vi "Finish.vi"   [LabVIEW 2015]
doc: "This VI is called just before exiting. It is expected to close I/O refnum, save collected data, etc."
uses:
  Robot Global.vi
  <vilib>/Rock Robotics/WPI/Ultrasonic/WPI_SonarMB1010AnalogClose.vi
types:
  T1 = typedef "Robot Drive.ctl" = cluster{"RobotDriveDevRef":T2, "Joysticks":cluster{"JoystickDevRef":T10, "JoystickDevRef 2":T10}, "Sensor":T12, "Pneumatics":T31, "Defenses":cluster{"LeftArm MotorControlDeviceRef":T3, "RightArm MotorControlDeviceRef":T3}, "Hanging":cluster{"Left Erection MotorControlDeviceRef":T3, "Right Erection MotorControlDeviceRef":T3}, "Aquisition + Scoring":T35, "DigitalOutputDevRef":T39, "DigitalInputDevRef":T16}
  T2 = typedef "WPI_RobotDriveDevRef.ctl" = cluster{"DevStatus":errorcluster, "Motors[]":T3[], "Square Inputs":bool, "Max Output":dbl}
  T3 = typedef "WPI_MotorControlDeviceRef.ctl" = cluster{"DeviceStatus":errorcluster, "Type":T4, "PWM":cluster{"PWM Channel":T5, "DeadBand":T6}, "CAN":cluster{"Device Number":u8, "Control Mode":T7, "Semaphore":T8, "Max Vout":dbl, "TalonSRX Control Mode":T9}, "Invert":bool}
  T4 = typedef "WPI_MotorControlType.ctl" = enum16{"PWM", "CAN", "CANTalonSRX"}
  T5 = typedef "FPGA_DIOPWMChannel.ctl" = enum8{"PWM 0", "PWM 1", "PWM 2", "PWM 3", "PWM 4", "PWM 5", "PWM 6", "PWM 7", "PWM 8", "PWM 9", "PWM MXP 0", "PWM MXP 1", "PWM MXP 2", "PWM MXP 3", "PWM MXP 4", "PWM MXP 5", "PWM MXP 6", "PWM MXP 7", "PWM MXP 8", "PWM MXP 9", "Invalid"}
  T6 = typedef "WPI_PWMDeadband.ctl" = cluster{"Name":string, "maxPositivePwm":i32, "minPositivePwm":i32, "centerPwm":i32, "maxNegativePwm":i32, "minNegativePwm":i32, "angularRange":u16}
  T7 = typedef "WPI_CANJaguar_ControlMode.ctl" = enum8{"Percent VBus", "Current", "Speed", "Position", "Voltage"}
  T8 = typedef "Semaphore RefNum" = refnum<k1>
  T9 = typedef "WPI_CANTalonSRX_APIControlMode.ctl" = enum8{"Percent VBus", "Speed", "Position", "Slave", "Unchanged / Invalid", "Voltage Compensation", "Current", "Motion Profile"}
  T10 = typedef "WPI_JoystickDevRef.ctl" = cluster{"Device":T11}
  T11 = typedef "WPI_JoystickDeviceEnum.ctl" = enum16{"USB 0", "USB 1", "USB 2", "USB 3", "USB 4", "USB 5"}
  T12 = typedef "Sensors.ctl" = cluster{"GyroDevRef":T13, "Left Arm Limit DigitalInputDevRef":T16, "Right Arm Limit DigitalInputDevRef":T16, "Left Arm EncoderDevRef":T18, "Right Arm EncoderDevRef":T18, "Left Drive EncoderDevRef":T18, "Right Drive EncoderDevRef":T18, "BoB Photoeye DigitalInputDevRef":T16, "Range SonarMB1010AnalogDevRef":T22, "Shooter CounterDevRef":T24, "AccelerometerDevRef":T25, "Left Hanging Erecter EncoderDevRef":T18, "Right Hanging Erecter EncoderDevRef":T18, "TestDigitalInputDevRef":T16, "Shooter Counter TopDevRef":T24}
  T13 = typedef "WPI_GyroDevRef.ctl" = cluster{"DevStatus":errorcluster, "Analog Channel":T14, "Offset":dbl, "Gain (VoltsPerDegree/Second)":dbl, "Gyro Type":enum16{"Analog", "XRS450"}, "Handle":i32, "SPI Bus":T15, "Device Found":bool, "Sample Rate":dbl, "Calibrate On Open":bool}
  T14 = typedef "FPGA_AIChannel.ctl" = enum8{"AI 0", "AI 1", "AI 2", "AI 3", "AI MXP 0", "AI MXP 1", "AI MXP 2", "AI MXP 3", "Invalid"}
  T15 = typedef "spi_bus.ctl" = enum16{"SPI On-Board, CS0", "SPI On-Board, CS1", "SPI On-Board, CS2", "SPI On-Board, CS3", "SPI MXP", "Invalid"}
  T16 = typedef "WPI_DigitalInputDevRef.ctl" = cluster{"DevStatus":errorcluster, "DIO Channel":T17}
  T17 = typedef "FPGA_DIOChannel.ctl" = enum8{"DIO 0", "DIO 1", "DIO 2", "DIO 3", "DIO 4", "DIO 5", "DIO 6", "DIO 7", "DIO 8", "DIO 9", "DIO MXP 0", "DIO MXP 1", "DIO MXP 2", "DIO MXP 3", "DIO MXP 4", "DIO MXP 5", "DIO MXP 6", "DIO MXP 7", "DIO MXP 8", "DIO MXP 9", "DIO MXP 10", "DIO MXP 11", "DIO MXP 12", "DIO MXP 13", "DIO MXP 14", "DIO MXP 15", "Invalid"}
  T18 = typedef "WPI_EncoderDevRef.ctl" = cluster{"DevStatus":errorcluster, "EncoderIndex":T19, "CounterIndex":T20, "DistancePerCount":dbl, "Decoding Type":T21}
  T19 = typedef "FPGA_EncoderIdx.ctl" = enum8{"Enc 0", "Enc 1", "Enc 2", "Enc 3", "Enc 4", "Enc 5", "Enc 6", "Enc 7", "Invalid"}
  T20 = typedef "FPGA_CounterCtrSystemIndex.ctl" = enum8{"Ctr 0", "Ctr 1", "Ctr 2", "Ctr 3", "Ctr 4", "Ctr 5", "Ctr 6", "Ctr 7", "Invalid"}
  T21 = typedef "WPI_EncoderType.ctl" = enum16{"1x", "2x", "4x"}
  T22 = typedef "WPI_SonarMB1010AnalogDeviceRef.ctl" = cluster{"AIDeviceRef":T23, "Scaling factor (V/in)":dbl, "Average Bits":u8}
  T23 = typedef "WPI_AnalogChannelDevRef.ctl" = cluster{"DevStatus":errorcluster, "Analog Channel":T14}
  T24 = typedef "WPI_CounterDevRef.ctl" = cluster{"DevStatus":errorcluster, "CntIndex":T20}
  T25 = typedef "WPI_AccelerometerDevRef.ctl" = cluster{"DevStatus":errorcluster, "Scaling":T26, "Analog Channels":T27, "I2C Bus":T28, "SPI Bus":T15, "Accel Range":T29, "ADXL Axes":T30, "Handle":i32, "Device Address":u8, "Accel Type":enum16{"Analog", "ADXL345 I2C", "ADXL345 SPI", "Internal", "ADXL362 SPI"}}
  T26 = typedef "WPI_AccelerometerScaling.ctl" = cluster{"Gain (VoltsPerG)":dbl, "Center Voltage":dbl}
  T27 = typedef "WPI_AccelerometerAnalogChannels.ctl" = cluster{"X-Axis":T14, "Y-Axis":T14, "Z-Axis":T14}
  T28 = typedef "i2c_bus.ctl" = enum16{"I2C On-Board", "I2C MXP", "Invalid"}
  T29 = typedef "ADXL345 Range.ctl" = u8
  T30 = typedef "WPI_AccelerometerADXL345 Axes.ctl" = cluster{"X-Axis":bool, "Y-Axis":bool, "Z-Axis":bool}
  T31 = typedef "Pnematics.ctl" = cluster{"CompressorDevRef":T32, "High and Low Gear DoubleSolenoidDevRef":T33, "PTO SolenoidDevRef":T33, "Hang Pin SolenoidDevRef":T33}
  T32 = typedef "WPI_CompressorDevRef.ctl" = cluster{"DevStatus":errorcluster, "Pneumatics Control Module":u8}
  T33 = typedef "WPI_SolenoidDevRef.ctl" = cluster{"DevStatus":errorcluster, "Pneumatics Control Module":u8, "Forward Solenoid Channel":T34, "Reverse Solenoid Channel":T34}
  T34 = typedef "WPI_SolenoidChannel.ctl" = enum8{"Solenoid 0", "Solenoid 1", "Solenoid 2", "Solenoid 3", "Solenoid 4", "Solenoid 5", "Solenoid 6", "Solenoid 7", "Invalid"}
  T35 = typedef "Acquisition & Scoring.ctl" = cluster{"Outer Roller MotorControlDeviceRef":T3, "Inner Roller MotorControlDeviceRef":T3, "Scoring Top MotorControlDeviceRef":T3, "Scoring Bottom MotorControlDeviceRef":T3, "Flashlight RelayDevRef":T36}
  T36 = typedef "WPI_RelayDevRef.ctl" = cluster{"DevStatus":errorcluster, "Relay Channel":T37, "Relay Direction":T38}
  T37 = typedef "FPGA_DIORelayChannel.ctl" = enum8{"Relay 0", "Relay 1", "Relay 2", "Relay 3", "Invalid"}
  T38 = typedef "WPI_RelayDirection.ctl" = enum16{"Both directions", "Forward only", "Reverse only"}
  T39 = typedef "WPI_DigitalOutputDevRef.ctl" = cluster{"DIO Channel":T17, "DevStatus":errorcluster}
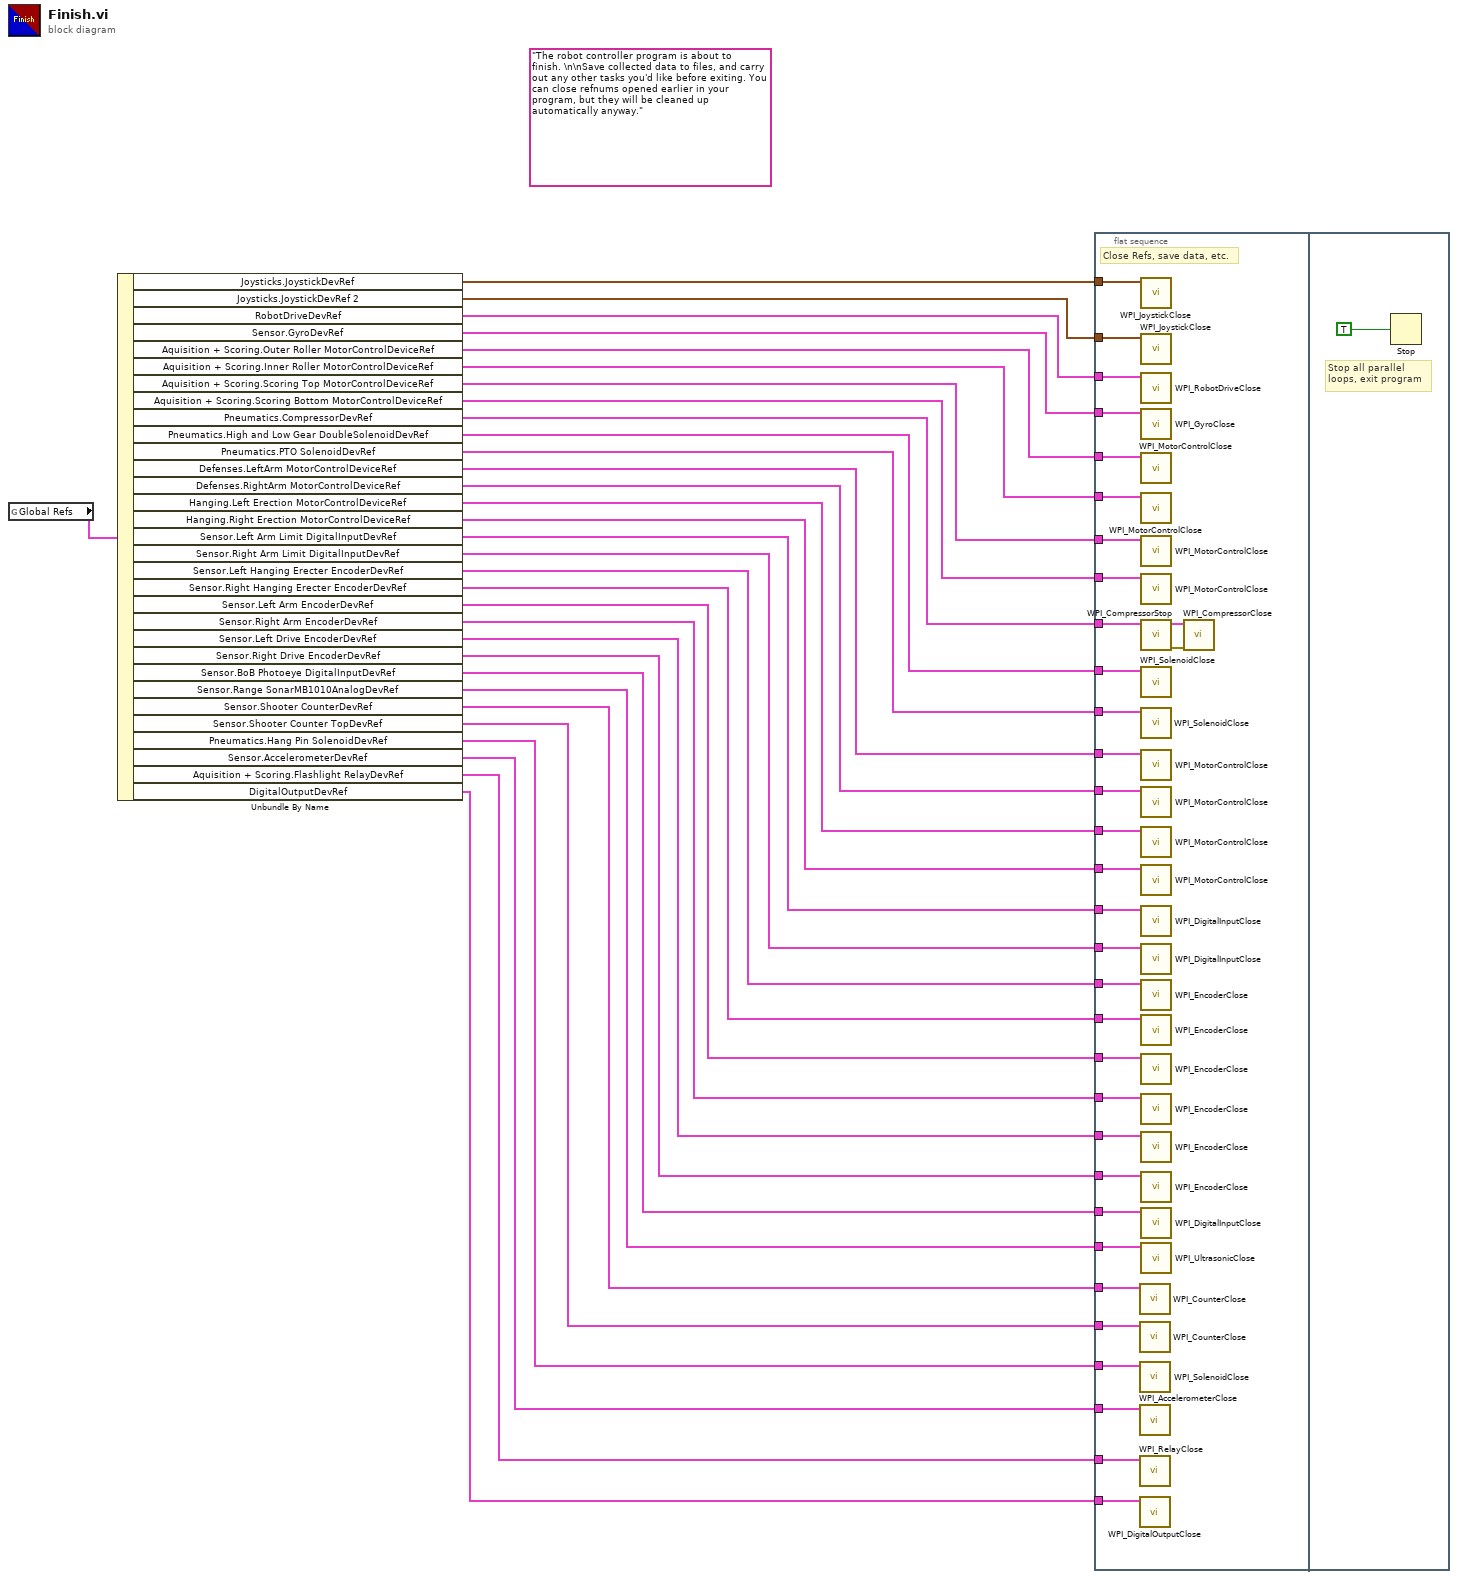
[diagram p0: block diagram]
diagram:
  (unwired) "The robot controller program is about to finish. \n\nSave collected data to files, and carry out any other tasks you'd like before exiting. You can close refnums opened earlier in your program, but they will be cleaned up automatically anyway."
  n1 = global read "Robot Global.vi" "Global Refs"() -> (w32:T1)
  n2 = Unbundle By Name(w32) -> ("Joysticks.JoystickDevRef"=w16:T10, "Joysticks.JoystickDevRef 2"=w17:T10, "RobotDriveDevRef"=w31:T2, "Sensor.GyroDevRef"=w30:T13, "Aquisition + Scoring.Outer Roller MotorControlDeviceRef"=w29:T3, "Aquisition + Scoring.Inner Roller MotorControlDeviceRef"=w6:T3, "Aquisition + Scoring.Scoring Top MotorControlDeviceRef"=w28:T3, "Aquisition + Scoring.Scoring Bottom MotorControlDeviceRef"=w27:T3, "Pneumatics.CompressorDevRef"=w26:T32, "Pneumatics.High and Low Gear DoubleSolenoidDevRef"=w25:T33, "Pneumatics.PTO SolenoidDevRef"=w24:T33, "Defenses.LeftArm MotorControlDeviceRef"=w23:T3, "Defenses.RightArm MotorControlDeviceRef"=w22:T3, "Hanging.Left Erection MotorControlDeviceRef"=w21:T3, "Hanging.Right Erection MotorControlDeviceRef"=w7:T3, "Sensor.Left Arm Limit DigitalInputDevRef"=w20:T16, "Sensor.Right Arm Limit DigitalInputDevRef"=w19:T16, "Sensor.Left Hanging Erecter EncoderDevRef"=w18:T18, "Sensor.Right Hanging Erecter EncoderDevRef"=w8:T18, "Sensor.Left Arm EncoderDevRef"=w15:T18, "Sensor.Right Arm EncoderDevRef"=w14:T18, "Sensor.Left Drive EncoderDevRef"=w13:T18, "Sensor.Right Drive EncoderDevRef"=w12:T18, "Sensor.BoB Photoeye DigitalInputDevRef"=w11:T16, "Sensor.Range SonarMB1010AnalogDevRef"=w10:T22, "Sensor.Shooter CounterDevRef"=w9:T24, "Sensor.Shooter Counter TopDevRef"=w1:T24, "Pneumatics.Hang Pin SolenoidDevRef"=w5:T33, "Sensor.AccelerometerDevRef"=w4:T25, "Aquisition + Scoring.Flashlight RelayDevRef"=w3:T36, "DigitalOutputDevRef"=w2:T39)
  n3 = flat-sequence {
    tunnel: w31 -> [w65]
    tunnel: w30 -> [w64]
    tunnel: w29 -> [w63]
    tunnel: w28 -> [w62]
    tunnel: w27 -> [w61]
    tunnel: w26 -> [w60]
    tunnel: w25 -> [w57]
    tunnel: w24 -> [w56]
    tunnel: w23 -> [w55]
    tunnel: w22 -> [w54]
    tunnel: w21 -> [w53]
    tunnel: w20 -> [w52]
    tunnel: w19 -> [w51]
    tunnel: w18 -> [w50]
    tunnel: w17 -> [w49]
    tunnel: w16 -> [w48]
    tunnel: w15 -> [w47]
    tunnel: w14 -> [w46]
    tunnel: w13 -> [w45]
    tunnel: w12 -> [w44]
    tunnel: w11 -> [w43]
    tunnel: w10 -> [w42]
    tunnel: w9 -> [w41]
    tunnel: w8 -> [w40]
    tunnel: w7 -> [w39]
    tunnel: w6 -> [w38]
    tunnel: w5 -> [w37]
    tunnel: w4 -> [w36]
    tunnel: w3 -> [w35]
    tunnel: w2 -> [w34]
    tunnel: w1 -> [w33]
    frame #0 {
      # "Close Refs, save data, etc."
      n4 = call <vilib>:"WPI_CounterClose.vi"("CounterDevRef"=w41) -> ()  [unwired: 10 in, 1 out]
      n5 = call <vilib>:"WPI_CounterClose.vi"("CounterDevRef"=w33) -> ()  [unwired: 10 in, 1 out]
      n6 = call <vilib>:"WPI_SolenoidClose.vi"("SolenoidDevRef"=w37) -> ()  [unwired: 10 in, 1 out]
      n7 = call <vilib>:"WPI_AccelerometerClose.vi"("AccelerometerDevRef"=w36) -> ()  [unwired: 10 in, 1 out]
      n8 = call <vilib>:"WPI_RelayClose.vi"("RelayDevRef"=w35) -> ()  [unwired: 10 in, 1 out]
      n9 = call <vilib>:"WPI_DigitalOutputClose.vi"("DigitalOutputDevRef"=w34) -> ()  [unwired: 10 in, 1 out]
      n10 = call <vilib>:"WPI_JoystickClose.vi"("JoystickDevRef"=w48) -> ()  [unwired: 11 out]
      n11 = call <vilib>:"WPI_JoystickClose.vi"("JoystickDevRef"=w49) -> ()  [unwired: 11 out]
      n12 = call <vilib>:"WPI_RobotDriveClose.vi"("RobotDriveDevRef"=w65) -> ()  [unwired: 1 in, 10 out]
      n13 = call <vilib>:"WPI_GyroClose.vi"("GyroDevRef"=w64) -> ()  [unwired: 10 in, 1 out]
      n14 = call <vilib>:"WPI_MotorControlClose.vi"("MotorControlDevRef"=w63) -> ()  [unwired: 10 in, 1 out]
      n15 = call <vilib>:"WPI_MotorControlClose.vi"("MotorControlDevRef"=w38) -> ()  [unwired: 10 in, 1 out]
      n16 = call <vilib>:"WPI_MotorControlClose.vi"("MotorControlDevRef"=w62) -> ()  [unwired: 10 in, 1 out]
      n17 = call <vilib>:"WPI_MotorControlClose.vi"("MotorControlDevRef"=w61) -> ()  [unwired: 10 in, 1 out]
      n18 = call <vilib>:"WPI_CompressorStop.vi"("CompressorDevRef"=w60) -> ("error out"=w59:errorcluster, "CompressorDevRef"=w58:T32)  [unwired: 9 in]
      n19 = call <vilib>:"WPI_SolenoidClose.vi"("SolenoidDevRef"=w57) -> ()  [unwired: 10 in, 1 out]
      n20 = call <vilib>:"WPI_SolenoidClose.vi"("SolenoidDevRef"=w56) -> ()  [unwired: 10 in, 1 out]
      n21 = call <vilib>:"WPI_MotorControlClose.vi"("MotorControlDevRef"=w55) -> ()  [unwired: 10 in, 1 out]
      n22 = call <vilib>:"WPI_MotorControlClose.vi"("MotorControlDevRef"=w54) -> ()  [unwired: 10 in, 1 out]
      n23 = call <vilib>:"WPI_MotorControlClose.vi"("MotorControlDevRef"=w53) -> ()  [unwired: 10 in, 1 out]
      n24 = call <vilib>:"WPI_MotorControlClose.vi"("MotorControlDevRef"=w39) -> ()  [unwired: 10 in, 1 out]
      n25 = call <vilib>:"WPI_DigitalInputClose.vi"("DigitalInputDevRef"=w52) -> ()  [unwired: 10 in, 1 out]
      n26 = call <vilib>:"WPI_DigitalInputClose.vi"("DigitalInputDevRef"=w51) -> ()  [unwired: 10 in, 1 out]
      n27 = call <vilib>:"WPI_EncoderClose.vi"("EncoderDevRef"=w50) -> ()  [unwired: 10 in, 1 out]
      n28 = call <vilib>:"WPI_EncoderClose.vi"("EncoderDevRef"=w40) -> ()  [unwired: 10 in, 1 out]
      n29 = call <vilib>:"WPI_EncoderClose.vi"("EncoderDevRef"=w47) -> ()  [unwired: 10 in, 1 out]
      n30 = call <vilib>:"WPI_EncoderClose.vi"("EncoderDevRef"=w46) -> ()  [unwired: 10 in, 1 out]
      n31 = call <vilib>:"WPI_EncoderClose.vi"("EncoderDevRef"=w45) -> ()  [unwired: 10 in, 1 out]
      n32 = call <vilib>:"WPI_EncoderClose.vi"("EncoderDevRef"=w44) -> ()  [unwired: 10 in, 1 out]
      n33 = call <vilib>:"WPI_DigitalInputClose.vi"("DigitalInputDevRef"=w43) -> ()  [unwired: 10 in, 1 out]
      n34 = call-poly <vilib>:"WPI_UltrasonicClose.vi"("SonarMB1010AnalogDevRef"=w42) -> ()  [unwired: 10 in, 1 out]
      n35 = call <vilib>:"WPI_CompressorClose.vi"("error in (no error)"=w59, "CompressorDevRef"=w58) -> ()  [unwired: 9 in, 1 out]
    }
    frame #1 {
      # "Stop all parallel\nloops, exit program"
      n36 = Stop(stop? (T)=TRUE ("Quit")) -> ()
    }
  }
